vi "GetTimeElements.vi"(1 "SECONDS":i32=123) -> (0 "String (relative time format)":string)   [LabVIEW 2015]
panel:
  out "I32 (relative time format)":i32 format="%<%H:%M:%S>t"
  out "Time Elements":i32[](array[numeric]) caption="H\nM\nS" format="%02d"
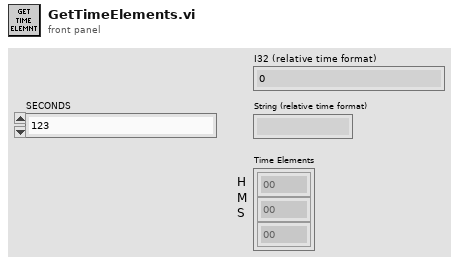
[diagram p1: front panel]
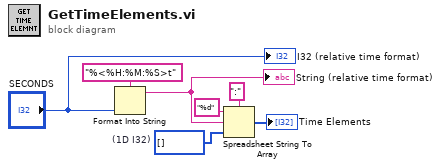
[diagram p0: block diagram]
diagram:
  w5 = i32[] []  # (1D I32)
  n1 = Format Into String(format string="%<%H:%M:%S>t", "SECONDS") -> (resulting string=w6:string)  [unwired: 2 in, 1 out]
  "String (relative time format)" <- w6
  n2 = Spreadsheet String To Array(delimiter (Tab)=":", format string="%d", spreadsheet string=w6, array type (2D Dbl)=w5) -> (array=→"Time Elements":i32[])
  "I32 (relative time format)" <- "SECONDS"
